vi "Diff_Drive_System_Begin.vi"   [LabVIEW 2019]
uses:
  <vilib>/Rock Robotics/SystemInterfaces/DIO/FPGA_DIOPWMChannel.ctl
  <vilib>/Rock Robotics/WPI/RobotDrive/WPI_RobotDriveOpen2MotorWithTalon.vi
  <vilib>/Rock Robotics/WPI/SafetyOutput/WPI_SafetyOutputConfigMenu.ctl
  <vilib>/Rock Robotics/SystemInterfaces/AI/FPGA_AIGyroChannel.ctl
  <vilib>/Rock Robotics/WPI/Counter/WPI_CounterDigitalInputToDigitalSource.vi
  <vilib>/Rock Robotics/SystemInterfaces/DIO/FPGA_DIOChannel.ctl
  <vilib>/Rock Robotics/WPI/Encoder/WPI_EncoderType.ctl
  <vilib>/Rock Robotics/WPI/Gyro/WPI_GyroAnalogOpen.vi
types:
  T1 = typedef "WPI_EncoderType.ctl" = enum16{"1x", "2x", "4x"}
  T2 = typedef "FPGA_DIOChannel.ctl" = enum8{"DIO 0", "DIO 1", "DIO 2", "DIO 3", "DIO 4", "DIO 5", "DIO 6", "DIO 7", "DIO 8", "DIO 9", "DIO MXP 0", "DIO MXP 1", "DIO MXP 2", "DIO MXP 3", "DIO MXP 4", "DIO MXP 5", "DIO MXP 6", "DIO MXP 7", "DIO MXP 8", "DIO MXP 9", "DIO MXP 10", "DIO MXP 11", "DIO MXP 12", "DIO MXP 13", "DIO MXP 14", "DIO MXP 15", "SPI Port CS1", "SPI Port CS2", "SPI Port CS3", "SPI Port MISO", "SPI Port MOSI", "Invalid"}
  T3 = typedef "WPI_SafetyOutputConfigMenu.ctl" = enum16{"Enable", "Disable"}
  T4 = typedef "FPGA_DIOPWMChannel.ctl" = enum8{"PWM 0", "PWM 1", "PWM 2", "PWM 3", "PWM 4", "PWM 5", "PWM 6", "PWM 7", "PWM 8", "PWM 9", "PWM MXP 0", "PWM MXP 1", "PWM MXP 2", "PWM MXP 3", "PWM MXP 4", "PWM MXP 5", "PWM MXP 6", "PWM MXP 7", "PWM MXP 8", "PWM MXP 9", "Invalid"}
  T5 = typedef "WPI_RobotDriveDevRef.ctl" = cluster{"DevStatus":errorcluster, "Motors[]":T6[], "Square Inputs":bool, "Max Output":dbl}
  T6 = typedef "WPI_MotorControlDeviceRef.ctl" = cluster{"DeviceStatus":errorcluster, "Type":T7, "PWM":cluster{"PWM Channel":T4, "DeadBand":T8}, "CAN":cluster{"Device Number":u8, "SetOutput VI Ref":variant, "GetOutput VI Ref":variant, "Enable VI Ref":variant, "Disable VI Ref":variant, "Data":variant}, "Invert":bool, "DIO PWM":cluster{"PWM \"Enable\" Channel":T4, "DIOChannel":T2, "PWM Rate":dbl}}
  T7 = typedef "WPI_MotorControlType.ctl" = enum16{"PWM", "CAN", "DIO PWM"}
  T8 = typedef "WPI_PWMDeadband.ctl" = cluster{"Name":string, "maxPositivePwm":i32, "minPositivePwm":i32, "centerPwm":i32, "maxNegativePwm":i32, "minNegativePwm":i32, "angularRange":u16}
  T9 = typedef "FPGA_AIGyroChannel.ctl" = enum8{"AI 0", "AI 1", "Invalid"}
  T10 = typedef "WPI_GyroDevRef.ctl" = cluster{"DevStatus":errorcluster, "Analog Channel":T11, "Gain (VoltsPerDegree/Second)":dbl, "Gyro Type":enum16{"Analog", "XRS450"}, "Handle":i32, "SPI Bus":T12, "Device Found":bool, "Sample Rate":dbl, "Calibrate On Open":bool, "Offset":dbl}
  T11 = typedef "FPGA_AIChannel.ctl" = enum8{"AI 0", "AI 1", "AI 2", "AI 3", "AI MXP 0", "AI MXP 1", "AI MXP 2", "AI MXP 3", "Invalid"}
  T12 = typedef "spi_bus.ctl" = enum16{"SPI On-Board, CS0", "SPI On-Board, CS1", "SPI On-Board, CS2", "SPI On-Board, CS3", "SPI MXP", "Invalid"}
  T13 = typedef "WPI_DigitalInputDevRef.ctl" = cluster{"DevStatus":errorcluster, "DIO Channel":T2}
  T14 = typedef "FPGA_CounterEncoderSourceConvertionLVSourceType.ctl" = cluster{"DevStatus":errorcluster, "AnalogTriggerMode?":bool, "DigitalMode":cluster{"DIO Channel":T15}, "AnalogTriggerMode":cluster{"AnalogTriggerIndex":T16, "OutputType":T17}}
  T15 = typedef "FPGA_DIODigitalSourceChannel.ctl" = enum8{"DIO 0", "DIO 1", "DIO 2", "DIO 3", "DIO 4", "DIO 5", "DIO 6", "DIO 7", "DIO 8", "DIO 9", "DIO MXP 0", "DIO MXP 1", "DIO MXP 2", "DIO MXP 3", "DIO MXP 4", "DIO MXP 5", "DIO MXP 6", "DIO MXP 7", "DIO MXP 8", "DIO MXP 9", "DIO MXP 10", "DIO MXP 11", "DIO MXP 12", "DIO MXP 13", "DIO MXP 14", "DIO MXP 15", "SPI Port CS1", "SPI Port CS2", "SPI Port CS3", "SPI Port MISO", "SPI Port MOSI", "Disabled"}
  T16 = typedef "FPGA_AnalogTriggerIndex.ctl" = enum8{"Trig 0", "Trig 1", "Trig 2", "Trig 3", "Trig 4", "Trig 5", "Trig 6", "Trig 7", "Invalid"}
  T17 = typedef "FPGA_AnalogTriggerOutType.ctl" = enum16{"InWindow", "TriggerState", "Rising", "Falling"}
  T18 = typedef "WPI_EncoderDevRef.ctl" = cluster{"DevStatus":errorcluster, "EncoderIndex":T19, "CounterIndex":T20, "DistancePerCount":dbl, "Decoding Type":T1}
  T19 = typedef "FPGA_EncoderIdx.ctl" = enum8{"Enc 0", "Enc 1", "Enc 2", "Enc 3", "Enc 4", "Enc 5", "Enc 6", "Enc 7", "Invalid"}
  T20 = typedef "FPGA_CounterCtrSystemIndex.ctl" = enum8{"Ctr 0", "Ctr 1", "Ctr 2", "Ctr 3", "Ctr 4", "Ctr 5", "Ctr 6", "Ctr 7", "Invalid"}
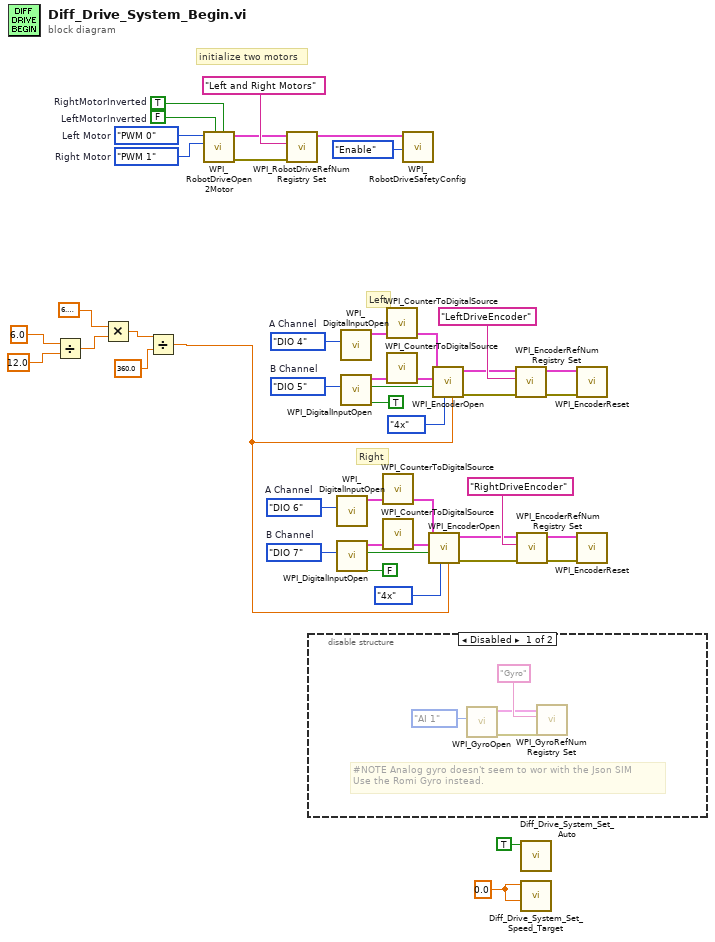
[diagram p0: block diagram]
diagram:
  w5 = 0.0 ("Left Speed Target FT/S")
  w24 = FPGA_DIOChannel."DIO 7"  # B Channel
  w25 = FPGA_DIOChannel."DIO 6"  # A Channel
  w28 = FPGA_DIOChannel."DIO 5"  # B Channel
  w29 = FPGA_DIOChannel."DIO 4"  # A Channel
  w13 = FPGA_DIOPWMChannel."PWM 1"  # Right Motor
  w12 = FPGA_DIOPWMChannel."PWM 0"  # Left Motor
  w8 = FALSE  # LeftMotorInverted
  w7 = TRUE  # RightMotorInverted
  # "Right"
  # "Left"
  # "initialize two motors"
  n1 = Divide(x=6.0, y=12.0) -> (x/y=w33:dbl)
  n2 = Multiply(x=6.283185307179586, y=w33) -> (x*y=w32:dbl)
  n3 = Divide(x=w32, y=360.0) -> (x/y=w38:dbl)
  n4 = call-poly <vilib>:"WPI_RobotDriveOpen2Motor.vi"("Right Motor Inverted"=w7, "Left Motor Inverted"=w8, "Right Motor"=w13, "Left Motor"=w12) -> ("error out"=w11:errorcluster, "RobotDriveDevRef"=w9:T5)  [unwired: 1 in, 5 out]
  n5 = call <vilib>:"WPI_RobotDriveRefNum Registry Set.vi"("error in (no error)"=w11, "refnum name"="Left and Right Motors", "RobotDriveDevRef"=w9) -> ("RobotDriveDevRef"=w14:T5)  [unwired: 1 in, 7 out]
  n6 = disable-structure shown="Disabled" {
    frame Disabled {
      # "#NOTE Analog gyro doesn't seem to wor with the Json SIM\nUse the Romi Gyro instead."
      n7 = call-poly <vilib>:"WPI_GyroOpen.vi"("Analog Channel"=FPGA_AIGyroChannel."AI 1") -> ("error out"=w46:errorcluster, "GyroDevRef"=w47:T10)  [unwired: 8 in, 1 out]
      n8 = call <vilib>:"WPI_GyroRefNum Registry Set.vi"("error in (no error)"=w46, "refnum name"="Gyro", "GyroDevRef"=w47) -> ()  [unwired: 7 in, 2 out]
    }
    frame Enabled {
    }
  }
  n9 = call <vilib>:"WPI_DigitalInputOpen.vi"("DIO Channel"=w25) -> ("DigitalInputDevRef"=w17:T13)  [unwired: 1 in, 9 out]
  n10 = call <vilib>:"WPI_DigitalInputOpen.vi"("DIO Channel"=w24) -> ("DigitalInputDevRef"=w18:T13)  [unwired: 1 in, 9 out]
  n11 = call <vilib>:"WPI_DigitalInputOpen.vi"("DIO Channel"=w29) -> ("DigitalInputDevRef"=w21:T13)  [unwired: 1 in, 9 out]
  n12 = call <vilib>:"WPI_DigitalInputOpen.vi"("DIO Channel"=w28) -> ("DigitalInputDevRef"=w22:T13)  [unwired: 1 in, 9 out]
  n13 = call-poly <vilib>:"WPI_CounterToDigitalSource.vi"("DigitalInputDevRef"=w17) -> ("Digital Source"=w16:T14)  [unwired: 6 out]
  n14 = call-poly <vilib>:"WPI_CounterToDigitalSource.vi"("DigitalInputDevRef"=w18) -> ("Digital Source"=w19:T14)  [unwired: 6 out]
  n15 = call-poly <vilib>:"WPI_CounterToDigitalSource.vi"("DigitalInputDevRef"=w21) -> ("Digital Source"=w20:T14)  [unwired: 6 out]
  n16 = call-poly <vilib>:"WPI_CounterToDigitalSource.vi"("DigitalInputDevRef"=w22) -> ("Digital Source"=w23:T14)  [unwired: 6 out]
  n17 = call <vilib>:"WPI_RobotDriveSafetyConfig.vi"("mode"=WPI_SafetyOutputConfigMenu."Enable", "RobotDriveDevRef"=w14) -> ()  [unwired: 8 in, 2 out]
  n18 = call <vilib>:"WPI_EncoderOpen.vi"("DistancePerCount"=w38, "Decoding Type"=WPI_EncoderType."4x", "Invert Direction (False)"=FALSE, "BSource"=w19, "ASource"=w16) -> ("error out"=w42:errorcluster, "EncoderDevRef"=w41:T18)  [unwired: 3 in, 2 out]
  n19 = call <vilib>:"WPI_EncoderOpen.vi"("DistancePerCount"=w38, "Decoding Type"=WPI_EncoderType."4x", "Invert Direction (False)"=TRUE, "BSource"=w23, "ASource"=w20) -> ("error out"=w40:errorcluster, "EncoderDevRef"=w39:T18)  [unwired: 3 in, 2 out]
  n20 = call <vilib>:"WPI_EncoderRefNum Registry Set.vi"("error in (no error)"=w40, "refnum name"="LeftDriveEncoder", "EncoderDevRef"=w39) -> ("error out"=w1:errorcluster, "EncoderDevRef"=w2:T18)  [unwired: 7 in]
  n21 = call <vilib>:"WPI_EncoderRefNum Registry Set.vi"("error in (no error)"=w42, "refnum name"="RightDriveEncoder", "EncoderDevRef"=w41) -> ("error out"=w4:errorcluster, "EncoderDevRef"=w3:T18)  [unwired: 7 in]
  n22 = call "Diff_Drive_System_Set_Auto.vi"("Auto Mode"=TRUE) -> ()  [unwired: 11 in]
  n23 = call "Diff_Drive_System_Set_Speed_Target.vi"("Right Speed Target FT/S"=w5, "Left Speed Target FT/S"=w5) -> ()  [unwired: 10 in]
  n24 = call <vilib>:"WPI_EncoderReset.vi"("error in (no error)"=w1, "EncoderDevRef"=w2) -> ()  [unwired: 8 in, 2 out]
  n25 = call <vilib>:"WPI_EncoderReset.vi"("error in (no error)"=w4, "EncoderDevRef"=w3) -> ()  [unwired: 8 in, 2 out]
